vi "Sample name judge.vi"(1 "Sample  Name:":string, 2 "START input":bool) -> (0 "START output":bool)   [LabVIEW 2011]
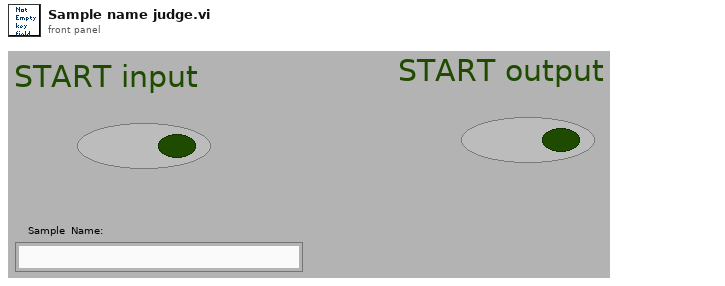
[diagram p1: front panel]
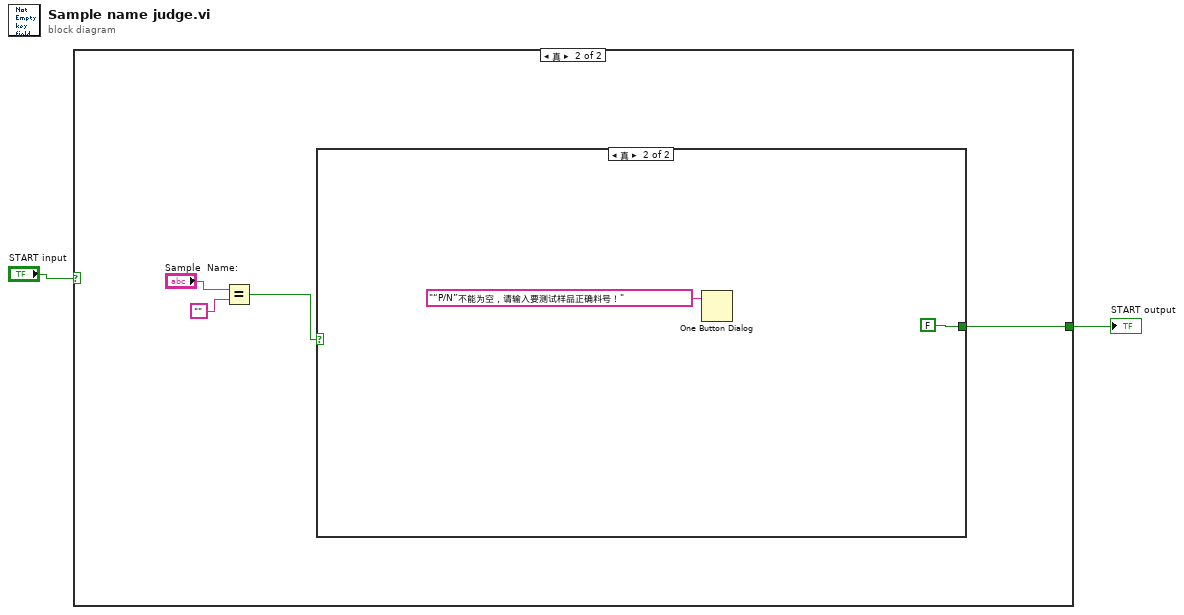
[diagram p0: block diagram]
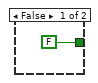
[diagram p2: hidden frame]
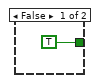
[diagram p3: hidden frame]
diagram:
  n1 = case shown="真" "START input" {
    tunnel: [FALSE ("START output") w6] -> w1
    frame False {
    }
    frame True {
      n2 = Equal?(x="Sample  Name:", y="") -> (x = y?=w7:bool)
      n3 = case shown="真" w7 {
        tunnel: [TRUE ("START output") FALSE ("START output")] -> w6
        frame False {
        }
        frame True {
          n4 = One Button Dialog(message="“P/N”不能为空，请输入要测试样品正确料号！") -> ()  [unwired: 1 in, 1 out]
        }
      }
    }
  }
  "START output" <- w1
